vi "snap_calibration_images.vi"(8 "error in (no error)":errorcluster, 10 "Number of Frames to Get":u32, 11 "Session In":T1) -> (0 "error out":errorcluster, 3 "Image Out":T2)   [LabVIEW 2019]
uses:
  <vilib>/vision/Image Controls.llb/IMAQ Image.ctl
  <vilib>/userDefined/High Color/IMAQdx.ctl
  <vilib>/vision/driver/IMAQdx.llb/IMAQdx Buffer Number Mode.ctl
  <vilib>/vision/driver/NI_Vision_Acquisition_Software.lvlib
  <vilib>/vision/NI_Vision_Development_Module.lvlib
panel:
  out "CameraBuffer Number":u32
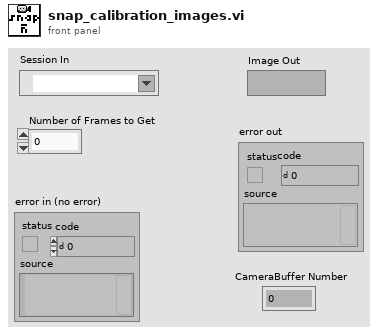
[diagram p1: front panel]
types:
  T1 = typedef "IMAQdx.ctl" = refnum<k21>
  T2 = typedef "IMAQ Image.ctl" = refnum<image>
  T3 = typedef "Image Type" = u32
  T4 = typedef "NI_Vision_Acquisition_Software.lvlib/IMAQdx Buffer Number Mode.ctl" = enum32{"Next", "Last", "Buffer Number", "Every", "Last New"}
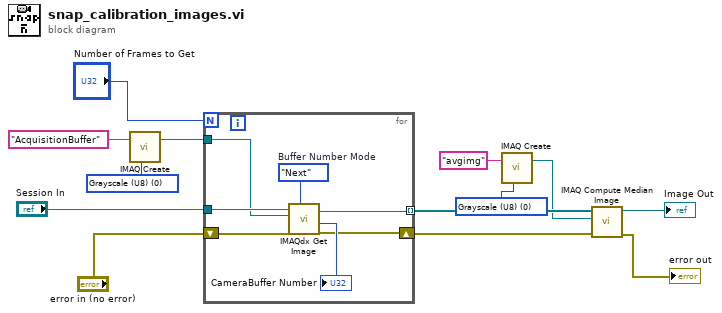
[diagram p0: block diagram]
diagram:
  w1 = T3 0 items=["Grayscale (U8)", "Grayscale (I16)", "Grayscale (SGL)", "Complex (CSG)", "RGB (U32)", "HSL (U32)", "RGB (U64)"] ("Image Type")
  w12 = T3 0 items=["Grayscale (U8)", "Grayscale (I16)", "Grayscale (SGL)", "Complex (CSG)", "RGB (U32)", "HSL (U32)", "RGB (U64)"] ("Image Type")
  n1 = call "IMAQ Create"("Image Name"="AcquisitionBuffer", "Image Type"=w12) -> ("New Image"=w11:T2)  [unwired: 3 in, 1 out]
  n2 = for {
    N: "Number of Frames to Get" -> [_]
    tunnel: w11 -> [w17]
    tunnel: "Session In" -> [w18]
    tunnel: [w15] -> w8 mode=indexing
    shift-right: [w14] -> w6
    shift-left: "error in (no error)" -> [w16]
    w20 = IMAQdx_Buffer_Number_Mode."Next"  # Buffer Number Mode
    n3 = call <vilib>:"IMAQdx Get Image.vi"("Buffer Number Mode (Next)"=w20, "error in"=w16, "Image In"=w17, "Session In"=w18) -> ("error out"=w14:errorcluster, "Buffer Number Out"=→"CameraBuffer Number":u32, "Image Out"=w15:T2)  [unwired: 4 in, 1 out]
  }
  n4 = call "IMAQ Create"("Image Name"="avgimg", "Image Type"=w1) -> ("New Image"=w3:T2)  [unwired: 3 in, 1 out]
  n5 = call "IMAQ Compute Median Image"("error in (no error)"=w6, "Image Dst"=w3, "Images"=w8) -> ("error out"=→"error out":errorcluster, "Image Dst Out"=→"Image Out":T2)  [unwired: 7 in]
